vi "Cartesian To Complex - RM,R.vi"(1 "Real Scalar k":dbl, 2 "Real Matrix R":T2) -> (0 "R + ki":T1)   [LabVIEW 2017, in "NI_Matrix.lvlib"]
doc: "Creates a complex number from two values in rectangular notation."
uses:
  NI_Matrix.lvlib
  RealMatrix.ctl
  ComplexMatrix.ctl
  Array To Matrix - CA2.vi
  Matrix To Array - RM.vi
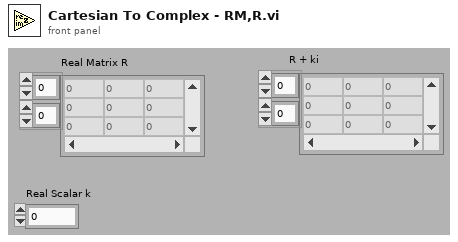
[diagram p1: front panel]
types:
  T1 = typedef "NI_Matrix.lvlib/ComplexMatrix.ctl" = cdb[][]
  T2 = typedef "NI_Matrix.lvlib/RealMatrix.ctl" = dbl[][]
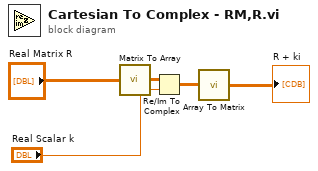
[diagram p0: block diagram]
diagram:
  n1 = call-poly "Matrix To Array.vi"("Real Matrix"="Real Matrix R") -> ("Real 2D Array"=w4:dbl[][])
  n2 = Re/Im To Complex(1:"Real Scalar k", 2:w4) -> (0:w2:cdb[][])
  n3 = call-poly "Array To Matrix.vi"("Complex 2D Array"=w2) -> ("Complex Matrix"=→"R + ki":T1)
